vi "PAM icListen Aquire AV TCP.vi"(3 "Acq In":T1, 4 "ID In":refnum<k5>, 5 "icListen #":i32) -> (0 "Acq Out":T1, 1 "Error Out":errorcluster)   [LabVIEW 2020]
uses:
  icListen 1 Synchronization.vi
  icListen 1 Response.vi
  icListen 2 Synchronization.vi
  icListen 2 Response.vi
  icListen 3 Synchronization.vi
  icListen 3 Response.vi
  icListen 4 Synchronization.vi
  icListen 4 Response.vi
  icListen 1 Connected.vi
  icListen 1 Initialized.vi
  icListen 2 Connected.vi
  icListen 2 Initialized.vi
  icListen 3 Connected.vi
  icListen 3 Initialized.vi
  icListen 4 Connected.vi
  icListen 4 Initialized.vi
  PAM Library.lvlib
panel:
  out "decimal integer string":string
  out "Notification":string
  out "Event Header":string
  out "Data Header":string
  in  "Error In":errorcluster
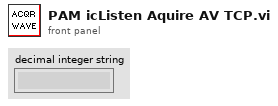
[diagram p1: front panel]
types:
  T1 = cluster{"State":enum16{"Align with Stream", "Read Header Byte", "Read Data Header", "Read Event Header", "Read Notification", "Read Data"}, "Sample Count":i32, "Timestamp":u64, "Payload":u16, "Repeated Error":i32, "Header Byte":string}
  T2 = enum16{"Align with Stream", "Read Header Byte", "Read Data Header", "Read Event Header", "Read Notification", "Read Data"}
  T3 = cluster{"default (0 U32)":i16, "Sample Count In":i32, "Timestamp In":u64}
  T4 = cluster{"State":enum16{"Align with Stream", "Read Header Byte", "Read Data Header", "Read Event Header", "Read Notification", "Read Data"}, i32, "Timestamp":u64, u16, i32, "substring":string}
  T5 = cluster{"State":enum16{"Align with Stream", "Read Header Byte", "Read Data Header", "Read Event Header", "Read Notification", "Read Data"}, "Sample Count":i32, "Timestamp":u64, u16, "Repeated Error":i32, "data out":string}
  T6 = cluster{"State":enum16{"Align with Stream", "Read Header Byte", "Read Data Header", "Read Event Header", "Read Notification", "Read Data"}, "Sample Count":i32, "Timestamp":u64, "Payload":u16, i32, "Header Byte":string}
  T7 = cluster{"State":enum16{"Align with Stream", "Read Header Byte", "Read Data Header", "Read Event Header", "Read Notification", "Read Data"}, "Sample Count":i32, "Timestamp":u64, i32, i32, "data out":string}
  T8 = cluster{"State":enum16{"Align with Stream", "Read Header Byte", "Read Data Header", "Read Event Header", "Read Notification", "Read Data"}, i32, "Timestamp":u64, "Payload":u16, "Repeated Error":i32, "data out":string}
  T9 = cluster{"State":enum16{"Align with Stream", "Read Header Byte", "Read Data Header", "Read Event Header", "Read Notification", "Read Data"}, "Sample Count":i32, "Timestamp":u64, "Payload":u16, "Repeated Error":i32, "data out":string}
  T10 = cluster{"default (0 U32)":i16, "Sample Count":i32, "Timestamp":u64}
  T11 = cluster{"State":enum16{"Align with Stream", "Read Header Byte", "Read Data Header", "Read Event Header", "Read Notification", "Read Data"}, "Sample Count":i32, "Timestamp":u64, "Payload":u16, i32, "data out":string}
  T12 = cluster{"System Time Status":u8, "Sync Status":u8, "PPS Count":u32, "Sync Offset":u32}
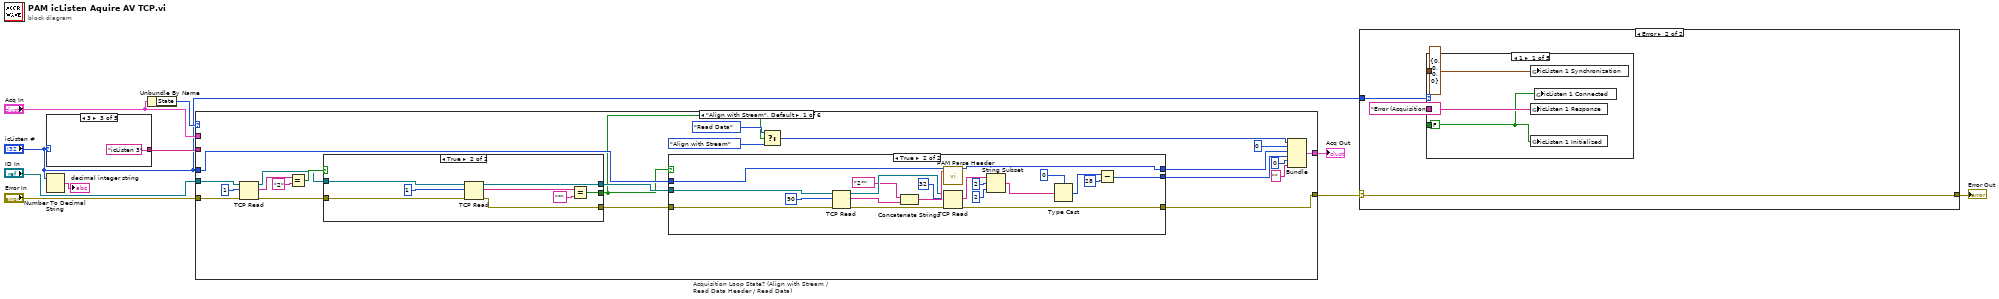
[diagram p0: block diagram]
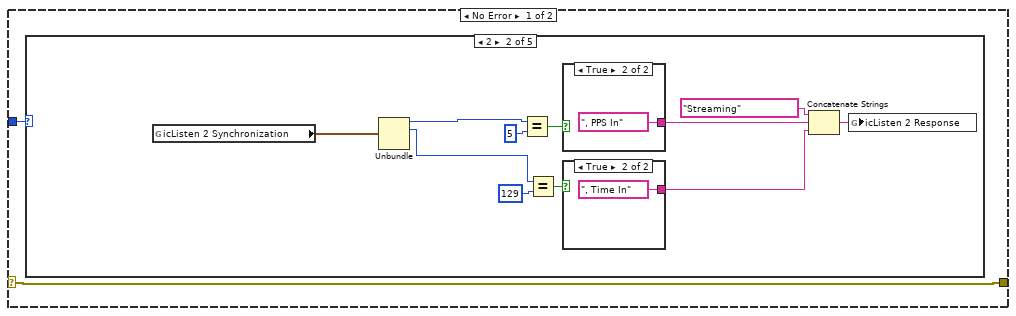
[diagram p2: hidden frame]
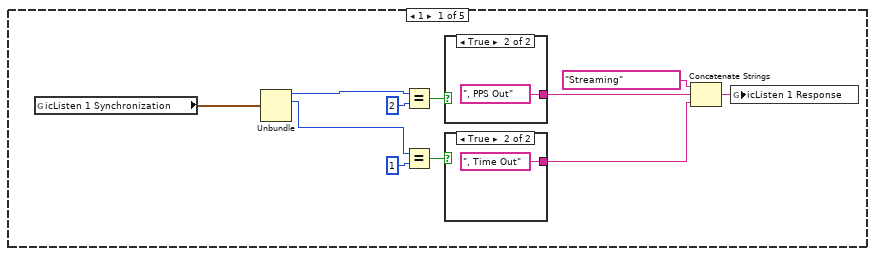
[diagram p3: hidden frame]
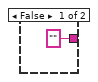
[diagram p4: hidden frame]
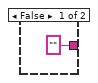
[diagram p5: hidden frame]
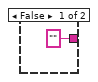
[diagram p6: hidden frame]
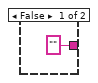
[diagram p7: hidden frame]
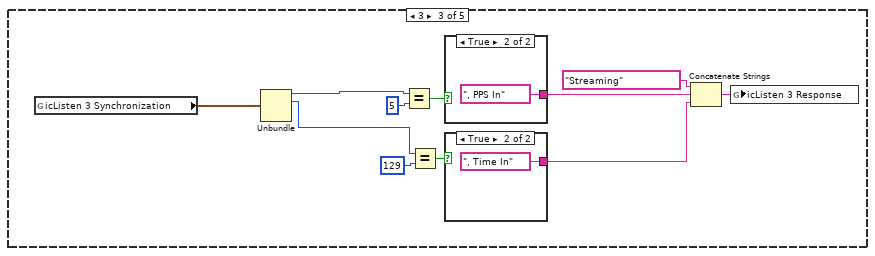
[diagram p8: hidden frame]
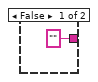
[diagram p9: hidden frame]
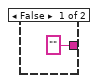
[diagram p10: hidden frame]
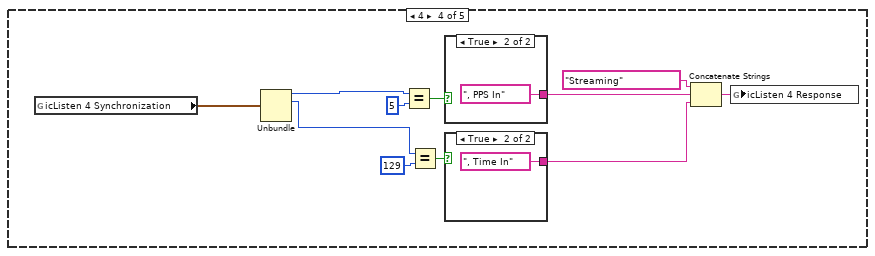
[diagram p11: hidden frame]
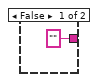
[diagram p12: hidden frame]
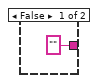
[diagram p13: hidden frame]
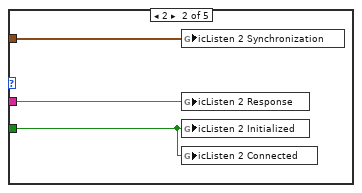
[diagram p15: hidden frame]
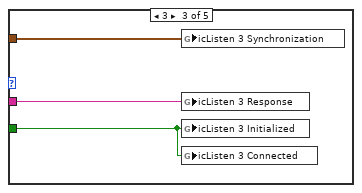
[diagram p16: hidden frame]
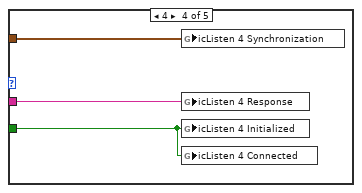
[diagram p17: hidden frame]
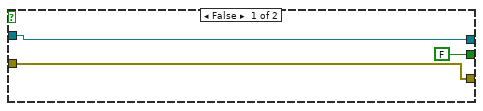
[diagram p19: hidden frame]
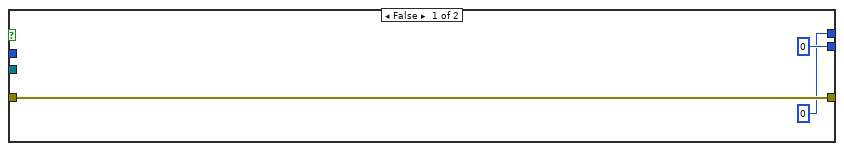
[diagram p20: hidden frame]
diagram:
  n1 = case shown="3" "icListen #" {
    tunnel: ["icListen 1" ("name (unnamed)") "icListen 2" ("name (unnamed)") "icListen 3" ("name (unnamed)") "icListen 4" ("name (unnamed)") _] -> w8
    frame 1 {
    }
    frame 2 {
    }
    frame 3 {
    }
    frame 4 {
    }
    frame 5, Default {
    }
  }
  n2 = Number To Decimal String(number="icListen #") -> (decimal integer string=→"decimal integer string":string)  [unwired: 1 in]
  n3 = Unbundle By Name("Acq In") -> ("State"=w5:T2)
  n4 = case "Acquisition Loop State? (Align with Stream / Read Data Header / Read Data)" shown="\"Align with Stream\", Default" w5 {
    selector: w5 -> [_ w76 _ _ _ _]
    tunnel: "Error In" -> [w34 w73 _ w161 w201 w249]
    tunnel: [w35 w72 w113 w159 w199 w244] -> w9
    tunnel: "icListen #" -> [w32 _ _ w156 w196 _]
    tunnel: w8 -> [_ _ _ _ _ w247]
    tunnel: "ID In" -> [w31 w71 w117 w162 w202 w246]
    tunnel: "Acq In" -> [_ w75 w114 w158 w198 w242]
    tunnel: [w24 w74 w116 w157 w197 w237] -> w6
    frame "Align with Stream", Default {
      n5 = TCP Read(connection ID=w31, bytes to read=1 ("byte count"), error in (no error)=w34) -> (connection ID out=w19:refnum<k5>, data out=w16:string, error out=w18:errorcluster)  [unwired: 2 in]
      n6 = Equal?(x=w16, y="2" ("x")) -> (x = y?=w21:bool)
      n7 = case shown="True" w21 {
        tunnel: [w39 w46] -> w20
        tunnel: w19 -> [w39 w45]
        tunnel: w18 -> [w38 w44]
        tunnel: [w38 w43] -> w17
        tunnel: [FALSE w40] -> w15
        frame False {
        }
        frame True {
          n8 = TCP Read(connection ID=w45, bytes to read=1 ("byte count"), error in (no error)=w44) -> (connection ID out=w46:refnum<k5>, data out=w42:string, error out=w43:errorcluster)  [unwired: 2 in]
          n9 = Equal?(x=w42, y="*" ("x")) -> (x = y?=w40:bool)
        }
      }
      n10 = case shown="True" w15 {
        tunnel: w17 -> [w50 w58]
        tunnel: [w50 w57] -> w35
        tunnel: [u16 0 w56] -> w30
        tunnel: [u64 0 ("Timestamp") w55] -> w29
        tunnel: w20 -> [_ w54]
        tunnel: w32 -> [_ w52]
        frame False {
        }
        frame True {
          n11 = TCP Read(connection ID=w54, bytes to read=90 ("byte count"), error in (no error)=w58) -> (connection ID out=w53:refnum<k5>, data out=w68:string, error out=w60:errorcluster)  [unwired: 2 in]
          n12 = Concatenate Strings("2*" ("x"), w68) -> (w69:string)
          n13 = call "PAM Parse Header.vi"("icListen #"=w52, "Header"=w69) -> ("Timestamp"=w55:u64)  [unwired: 17 in]
          n14 = TCP Read(connection ID=w53, bytes to read=32 ("byte count"), error in (no error)=w60) -> (data out=w70:string, error out=w57:errorcluster)  [unwired: 2 in, 1 out]
          n15 = String Subset(string=w70, offset (0)=2, length (rest)=2 ("length (rest)")) -> (substring=w63:string)
          n16 = Type Cast(type=u16 0, x=w63) -> (*(type *) &x=w67:u16)
          n17 = Subtract(x=w67, y=u16 28 ("x")) -> (x-y=w56:u16)
        }
      }
      n18 = Select(t=T2."Read Data" ("State"), s=w15, f=T2."Align with Stream" ("State")) -> (s? t:f=w27:T2)
      n19 = Bundle("State"=w27, 0, "Timestamp"=w29, w30, 0, "substring"="") -> (w24:T4)  [unwired: 1 in]
    }
    frame "Read Header Byte" {
      n20 = TCP Read(connection ID=w71, bytes to read=2 ("byte count"), error in (no error)=w73, 9:0 ("timeout ms (25000)")) -> (connection ID out=w79:refnum<k5>, data out=w81:string, error out=w80:errorcluster)  [unwired: 1 in]
      n21 = Type Cast(type=u16 0, x=w81) -> (*(type *) &x=w83:u16)
      n22 = case shown="No Error" w80 {
        selector: w80 -> [w92 w107]
        tunnel: w83 -> [w90 _]
        tunnel: w81 -> [w91 _]
        tunnel: [w92 w108] -> w72
        tunnel: w76 -> [_ _]
        tunnel: w79 -> [_ _]
        tunnel: w75 -> [w86 w105]
        tunnel: [w87 w97] -> w74
        frame No Error {
          w88 = 0  # Repeated Error
          n23 = case shown="12586" w90 {
            tunnel: [w93 w94 w95 _] -> w89
            frame 12586 {
              w93 = T2."Read Data Header"  # State
              # "Data Header"
            }
            frame 12842 {
              w94 = T2."Read Event Header"  # State
              # "Event Header"
            }
            frame 12330 {
              w95 = T2."Read Notification"  # State
              # "Notification"
            }
            frame 0, Default {
            }
          }
          n24 = Unbundle(w86) -> ("Sample Count"=w85:i32, "Timestamp"=w84:u64)  [unwired: 4 out]
          n25 = Bundle("State"=w89, "Sample Count"=w85, "Timestamp"=w84, w90, "Repeated Error"=w88, "data out"=w91) -> (w87:T5)  [unwired: 1 in]
        }
        frame Error {
          n26 = Unbundle(w105) -> ("State"=w104:T2, "Sample Count"=w103:i32, "Timestamp"=w102:u64, "Payload"=w101:u16, "Repeated Error"=w98:i32, "Header Byte"=w100:string)
          n27 = Add(x=w98, y=1) -> (x+y=w99:i32)
          n28 = Equal?(x=w98, y=100000) -> (x = y?=w109:bool)
          n29 = Bundle("State"=w104, "Sample Count"=w103, "Timestamp"=w102, "Payload"=w101, w99, "Header Byte"=w100) -> (w97:T6)  [unwired: 1 in]
          n30 = case shown="True" w109 {
            tunnel: [errorcluster {"status"=FALSE, "code"=0, "source"=""} ("error IO") w112] -> w108
            tunnel: w107 -> [_ w112]
            frame False {
            }
            frame True {
            }
          }
          n31 = Wait (ms)(milliseconds to wait=u32 2) -> ()  [unwired: 1 out]
        }
      }
    }
    frame "Read Data Header" {
      n32 = TCP Read(connection ID=w117, bytes to read=30 ("byte count"), 9:0 ("timeout ms (25000)")) -> (data out=w119:string, error out=w115:errorcluster)  [unwired: 2 in, 1 out]
      n33 = case shown="No Error" w115 {
        selector: w115 -> [w127 w140]
        tunnel: w119 -> [w131 _]
        tunnel: [w122 w142] -> w116
        tunnel: w114 -> [w125 w143]
        tunnel: [w127 w141] -> w113
        frame No Error {
          w126 = T2."Read Data"  # State
          n34 = Unbundle(w125) -> ("Sample Count"=w124:i32, "Timestamp"=w123:u64, "Header Byte"=w121:string)  [unwired: 3 out]
          n35 = Concatenate Strings(w121, w131) -> (w132:string)
          n36 = String Subset(string=w132, offset (0)=2, length (rest)=2 ("length (rest)")) -> (substring=w137:string)
          n37 = Type Cast(type=u16 0, x=w137) -> (*(type *) &x=w134:u16)
          n38 = Subtract(x=w134, y=28 ("x")) -> (x-y=w130:i32)
          n39 = Bundle("State"=w126, "Sample Count"=w124, "Timestamp"=w123, w130, 0, "data out"="") -> (w122:T7)  [unwired: 1 in]
          "Data Header" <- w131
        }
        frame Error {
          n40 = Unbundle(w143) -> ("State"=w150:T2, "Sample Count"=w149:i32, "Timestamp"=w148:u64, "Payload"=w147:u16, "Repeated Error"=w144:i32, "Header Byte"=w146:string)
          n41 = Add(x=w144, y=1) -> (x+y=w145:i32)
          n42 = Equal?(x=w144, y=100000) -> (x = y?=w152:bool)
          n43 = Bundle("State"=w150, "Sample Count"=w149, "Timestamp"=w148, "Payload"=w147, w145, "Header Byte"=w146) -> (w142:T6)  [unwired: 1 in]
          n44 = case shown="True" w152 {
            tunnel: [errorcluster {"status"=FALSE, "code"=0, "source"=""} ("error IO") w155] -> w141
            tunnel: w140 -> [_ w155]
            frame False {
            }
            frame True {
            }
          }
          n45 = Wait (ms)(milliseconds to wait=u32 2) -> ()  [unwired: 1 out]
        }
      }
    }
    frame "Read Event Header" {
      n46 = TCP Read(connection ID=w162, bytes to read=90 ("byte count"), error in (no error)=w161, 9:0 ("timeout ms (25000)")) -> (data out=w164:string, error out=w160:errorcluster)  [unwired: 1 in, 1 out]
      n47 = case shown="No Error" w160 {
        selector: w160 -> [w173 w183]
        tunnel: w164 -> [w178 _]
        tunnel: [w173 w182] -> w159
        tunnel: w158 -> [w176 w181]
        tunnel: [w174 w180] -> w157
        tunnel: w156 -> [w168 _]
        frame No Error {
          w175 = T2."Read Header Byte"  # State
          n48 = Unbundle(w176) -> ("Header Byte"=w169:string)  [unwired: 5 out]
          n49 = Concatenate Strings(w169, w178) -> (w177:string)
          n50 = call "PAM Parse Header.vi"("icListen #"=w168, "Header"=w177) -> ("Timestamp"=w167:u64)  [unwired: 17 in]
          n51 = Bundle("State"=w175, 0, "Timestamp"=w167, "Payload"=u16 0, "Repeated Error"=0, "data out"="") -> (w174:T8)  [unwired: 1 in]
          "Event Header" <- w178
        }
        frame Error {
          n52 = Unbundle(w181) -> ("State"=w190:T2, "Sample Count"=w189:i32, "Timestamp"=w188:u64, "Payload"=w187:u16, "Repeated Error"=w184:i32, "Header Byte"=w186:string)
          n53 = Add(x=w184, y=1) -> (x+y=w185:i32)
          n54 = Equal?(x=w184, y=100000) -> (x = y?=w192:bool)
          n55 = Bundle("State"=w190, "Sample Count"=w189, "Timestamp"=w188, "Payload"=w187, w185, "Header Byte"=w186) -> (w180:T6)  [unwired: 1 in]
          n56 = case shown="True" w192 {
            tunnel: [errorcluster {"status"=FALSE, "code"=0, "source"=""} ("error IO") w195] -> w182
            tunnel: w183 -> [_ w195]
            frame False {
            }
            frame True {
            }
          }
          n57 = Wait (ms)(milliseconds to wait=u32 2) -> ()  [unwired: 1 out]
        }
      }
    }
    frame "Read Notification" {
      n58 = TCP Read(connection ID=w202, bytes to read=6 ("byte count"), error in (no error)=w201, 9:0 ("timeout ms (25000)")) -> (data out=w204:string, error out=w200:errorcluster)  [unwired: 1 in, 1 out]
      n59 = case shown="No Error" w200 {
        selector: w200 -> [w213 w223]
        tunnel: w204 -> [w218 _]
        tunnel: [w213 w222] -> w199
        tunnel: w198 -> [w216 w221]
        tunnel: [w206 w220] -> w197
        tunnel: w196 -> [w208 _]
        frame No Error {
          w215 = T2."Read Header Byte"  # State
          n60 = Unbundle(w216) -> ("Sample Count"=w214:i32, "Header Byte"=w209:string)  [unwired: 4 out]
          n61 = Concatenate Strings(w209, w218) -> (w217:string)
          n62 = call "PAM Parse Header.vi"("icListen #"=w208, "Header"=w217) -> ("Timestamp"=w207:u64)  [unwired: 17 in]
          n63 = Bundle("State"=w215, "Sample Count"=w214, "Timestamp"=w207, "Payload"=u16 0, "Repeated Error"=0, "data out"="") -> (w206:T9)  [unwired: 1 in]
          "Notification" <- w218
        }
        frame Error {
          n64 = Unbundle(w221) -> ("State"=w230:T2, "Sample Count"=w229:i32, "Timestamp"=w228:u64, "Payload"=w227:u16, "Repeated Error"=w224:i32, "Header Byte"=w226:string)
          n65 = Add(x=w224, y=1) -> (x+y=w225:i32)
          n66 = Equal?(x=w224, y=100000) -> (x = y?=w232:bool)
          n67 = Bundle("State"=w230, "Sample Count"=w229, "Timestamp"=w228, "Payload"=w227, w225, "Header Byte"=w226) -> (w220:T6)  [unwired: 1 in]
          n68 = case shown="True" w232 {
            tunnel: [errorcluster {"status"=FALSE, "code"=0, "source"=""} ("error IO") w235] -> w222
            tunnel: w223 -> [_ w235]
            frame False {
            }
            frame True {
            }
          }
          n69 = Wait (ms)(milliseconds to wait=u32 2) -> ()  [unwired: 1 out]
        }
      }
    }
    frame "Read Data" {
      n70 = Unbundle(w242) -> ("State"=w236:T2, "Sample Count"=w241:i32, "Timestamp"=w240:u64, "Payload"=w239:u16, "Repeated Error"=w238:i32)  [unwired: 1 out]
      n71 = TCP Read(connection ID=w246, bytes to read=w239, error in (no error)=w249, 9:0 ("timeout ms (25000)")) -> (data out=w248:string, error out=w243:errorcluster)  [unwired: 1 in, 1 out]
      n72 = case shown="No Error" w243 {
        selector: w243 -> [w257 w289]
        tunnel: w248 -> [w269 _]
        tunnel: w241 -> [w268 w284]
        tunnel: w240 -> [w254 w283]
        tunnel: w247 -> [w267 _]
        tunnel: [w258 w287] -> w244
        tunnel: w239 -> [_ w282]
        tunnel: w238 -> [_ w288]
        tunnel: [w250 w286] -> w237
        tunnel: w236 -> [_ w285]
        frame No Error {
          w256 = T2."Read Header Byte"  # State
          n73 = Type Cast(type=i16[] [], x=w269) -> (*(type *) &x=w265:i16[])
          n74 = Obtain Queue(name (unnamed)=w267, element data type=T3 {"default (0 U32)"=0, "Sample Count In"=0, "Timestamp In"=0} ("output cluster"), create if not found? (T)=FALSE, error in (no error)=w257) -> (queue out=w261:refnum<queue>, error out=w264:errorcluster)  [unwired: 1 in, 1 out]
          n75 = for {
            tunnel: w265 -> [w278] mode=indexing
            shift-right: [w274] -> w255
            shift-left: w268 -> [w275]
            tunnel: w254 -> [w277]
            tunnel: w264 -> [w273]
            tunnel: [w272] -> w263
            tunnel: w261 -> [w271]
            tunnel: [w270] -> w259
            n76 = Increment(x=w275) -> (x+1=w274:i32)
            n77 = Bundle("default (0 U32)"=w278, "Sample Count"=w275, "Timestamp"=w277) -> (w276:T10)  [unwired: 1 in]
            n78 = Lossy Enqueue Element(queue=w271, element=w276, error in (no error)=w273) -> (queue out=w270:refnum<queue>, error out=w272:errorcluster)  [unwired: 2 out]
          }
          n79 = Release Queue(queue=w259, error in (no error)=w263) -> (error out=w258:errorcluster)  [unwired: 1 in, 2 out]
          n80 = Bundle("State"=w256, "Sample Count"=w255, "Timestamp"=w254, 0, 0, "data out"="") -> (w250:T7)  [unwired: 1 in]
        }
        frame Error {
          n81 = Add(x=w288, y=1) -> (x+y=w281:i32)
          n82 = Equal?(x=w288, y=100000) -> (x = y?=w291:bool)
          n83 = Bundle("State"=w285, "Sample Count"=w284, "Timestamp"=w283, "Payload"=w282, w281, "data out"="") -> (w286:T11)  [unwired: 1 in]
          n84 = case shown="True" w291 {
            tunnel: [errorcluster {"status"=FALSE, "code"=0, "source"=""} ("error IO") w294] -> w287
            tunnel: w289 -> [_ w294]
            frame False {
            }
            frame True {
            }
          }
          n85 = Wait (ms)(milliseconds to wait=u32 2) -> ()  [unwired: 1 out]
        }
      }
    }
  }
  "Acq Out" <- w6
  n86 = case shown="Error" w9 {
    selector: w9 -> [w295 w357]
    tunnel: "icListen #" -> [w296 w358]
    tunnel: [w295 w357] -> w3
    frame No Error {
      n87 = case shown="2" w296 {
        frame 1 {
          n88 = global read "icListen 1 Synchronization.vi" "icListen 1 Synchronization"() -> (w303:T12)
          n89 = Unbundle(w303) -> ("System Time Status"=w305:u8, "Sync Status"=w307:u8)  [unwired: 2 out]
          n90 = Equal?(x=w305, y=u8 2) -> (x = y?=w302:bool)
          n91 = Equal?(x=w307, y=u8 1) -> (x = y?=w301:bool)
          n92 = case shown="True" w302 {
            tunnel: ["" ("icListen 2 Response 2") ", PPS Out" ("icListen 2 Response 2")] -> w299
            frame False {
            }
            frame True {
            }
          }
          n93 = case shown="True" w301 {
            tunnel: ["" ("icListen 2 Response 2") ", Time Out" ("icListen 2 Response 2")] -> w298
            frame False {
            }
            frame True {
            }
          }
          n94 = Concatenate Strings("Streaming" ("icListen 2 Response 2"), w299, w298) -> (w297:string)
          n95 = global write "icListen 1 Response.vi" "icListen 1 Response"(w297) -> ()
        }
        frame 2 {
          n96 = global read "icListen 2 Synchronization.vi" "icListen 2 Synchronization"() -> (w313:T12)
          n97 = Unbundle(w313) -> ("System Time Status"=w320:u8, "Sync Status"=w322:u8)  [unwired: 2 out]
          n98 = Equal?(x=w320, y=u8 5) -> (x = y?=w318:bool)
          n99 = Equal?(x=w322, y=u8 129) -> (x = y?=w317:bool)
          n100 = case shown="True" w318 {
            tunnel: ["" ("icListen 2 Response 2") ", PPS In" ("icListen 2 Response 2")] -> w315
            frame False {
            }
            frame True {
            }
          }
          n101 = case shown="True" w317 {
            tunnel: ["" ("icListen 2 Response 2") ", Time In" ("icListen 2 Response 2")] -> w314
            frame False {
            }
            frame True {
            }
          }
          n102 = Concatenate Strings("Streaming" ("icListen 2 Response 2"), w315, w314) -> (w312:string)
          n103 = global write "icListen 2 Response.vi" "icListen 2 Response"(w312) -> ()
        }
        frame 3 {
          n104 = global read "icListen 3 Synchronization.vi" "icListen 3 Synchronization"() -> (w328:T12)
          n105 = Unbundle(w328) -> ("System Time Status"=w335:u8, "Sync Status"=w337:u8)  [unwired: 2 out]
          n106 = Equal?(x=w335, y=u8 5) -> (x = y?=w333:bool)
          n107 = Equal?(x=w337, y=u8 129) -> (x = y?=w332:bool)
          n108 = case shown="True" w333 {
            tunnel: ["" ("icListen 2 Response 2") ", PPS In" ("icListen 2 Response 2")] -> w330
            frame False {
            }
            frame True {
            }
          }
          n109 = case shown="True" w332 {
            tunnel: ["" ("icListen 2 Response 2") ", Time In" ("icListen 2 Response 2")] -> w329
            frame False {
            }
            frame True {
            }
          }
          n110 = Concatenate Strings("Streaming" ("icListen 2 Response 2"), w330, w329) -> (w327:string)
          n111 = global write "icListen 3 Response.vi" "icListen 3 Response"(w327) -> ()
        }
        frame 4 {
          n112 = global read "icListen 4 Synchronization.vi" "icListen 4 Synchronization"() -> (w342:T12)
          n113 = Unbundle(w342) -> ("System Time Status"=w350:u8, "Sync Status"=w352:u8)  [unwired: 2 out]
          n114 = Equal?(x=w350, y=u8 5) -> (x = y?=w348:bool)
          n115 = Equal?(x=w352, y=u8 129) -> (x = y?=w347:bool)
          n116 = case shown="True" w348 {
            tunnel: ["" ("icListen 2 Response 2") ", PPS In" ("icListen 2 Response 2")] -> w345
            frame False {
            }
            frame True {
            }
          }
          n117 = case shown="True" w347 {
            tunnel: ["" ("icListen 2 Response 2") ", Time In" ("icListen 2 Response 2")] -> w344
            frame False {
            }
            frame True {
            }
          }
          n118 = Concatenate Strings("Streaming" ("icListen 2 Response 2"), w345, w344) -> (w343:string)
          n119 = global write "icListen 4 Response.vi" "icListen 4 Response"(w343) -> ()
        }
        frame 5, Default {
        }
      }
    }
    frame Error {
      n120 = case shown="1" w358 {
        tunnel: FALSE -> [w362 w366 w369 w372 _]
        tunnel: "Error (Acquisition)" ("icListen 2 Response 2") -> [w364 w367 w370 w373 _]
        tunnel: T12 {"System Time Status"=0, "Sync Status"=0, "PPS Count"=0, "Sync Offset"=0} ("icListen 1 Synchronization") -> [w363 w365 w368 w371 _]
        frame 1 {
          n121 = global write "icListen 1 Synchronization.vi" "icListen 1 Synchronization"(w363) -> ()
          n122 = global write "icListen 1 Response.vi" "icListen 1 Response"(w364) -> ()
          n123 = global write "icListen 1 Initialized.vi" "icListen 1 Initialized"(w362) -> ()
          n124 = global write "icListen 1 Connected.vi" "icListen 1 Connected"(w362) -> ()
        }
        frame 2 {
          n125 = global write "icListen 2 Synchronization.vi" "icListen 2 Synchronization"(w365) -> ()
          n126 = global write "icListen 2 Response.vi" "icListen 2 Response"(w367) -> ()
          n127 = global write "icListen 2 Initialized.vi" "icListen 2 Initialized"(w366) -> ()
          n128 = global write "icListen 2 Connected.vi" "icListen 2 Connected"(w366) -> ()
        }
        frame 3 {
          n129 = global write "icListen 3 Synchronization.vi" "icListen 3 Synchronization"(w368) -> ()
          n130 = global write "icListen 3 Response.vi" "icListen 3 Response"(w370) -> ()
          n131 = global write "icListen 3 Initialized.vi" "icListen 3 Initialized"(w369) -> ()
          n132 = global write "icListen 3 Connected.vi" "icListen 3 Connected"(w369) -> ()
        }
        frame 4 {
          n133 = global write "icListen 4 Synchronization.vi" "icListen 4 Synchronization"(w371) -> ()
          n134 = global write "icListen 4 Response.vi" "icListen 4 Response"(w373) -> ()
          n135 = global write "icListen 4 Initialized.vi" "icListen 4 Initialized"(w372) -> ()
          n136 = global write "icListen 4 Connected.vi" "icListen 4 Connected"(w372) -> ()
        }
        frame 5, Default {
        }
      }
    }
  }
  "Error Out" <- w3
